vi "Validate Rate.vi"(8 "error IO":errorcluster, 9 "Ramping Mode":T1, 10 "rate":dbl[unit] caption="Rate", 11 "Power Supply in":refnum<class "Power Supply.lvclass">) -> (0 "error out":errorcluster, 1 "Max rate":dbl[unit], 2 "Coerced rate":dbl[unit], 3 "Power Supply out":refnum<class "Power Supply.lvclass">, 4 "Coerced?":bool, 6 "Field":dbl[unit])   [LabVIEW 2009, in "Power Supply.lvclass"]
doc: "Query the current field and verify that the given sweep rate is appropriate for this field."
uses:
  Power Supply.lvclass
  Ramping Mode.ctl
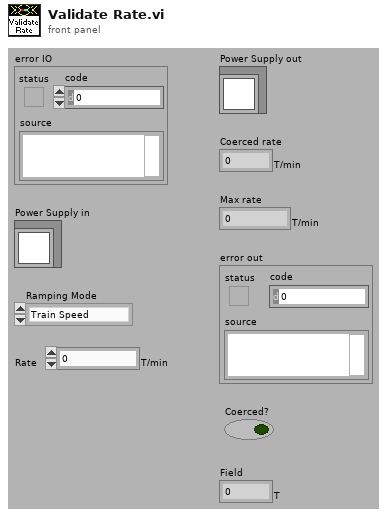
[diagram p1: front panel]
types:
  T1 = typedef "Power Supply.lvclass/Ramping Mode.ctl" = enum16{"Train Speed", "Maximum Speed", "Manual"}
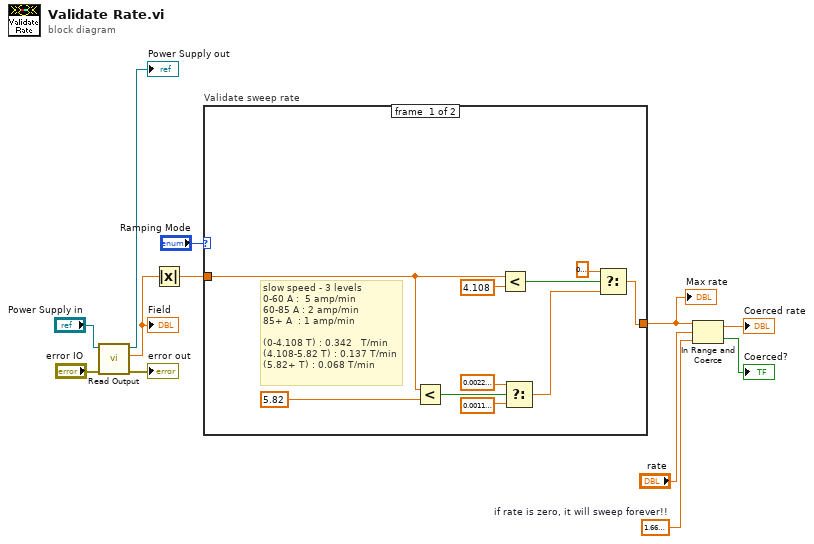
[diagram p0: block diagram]
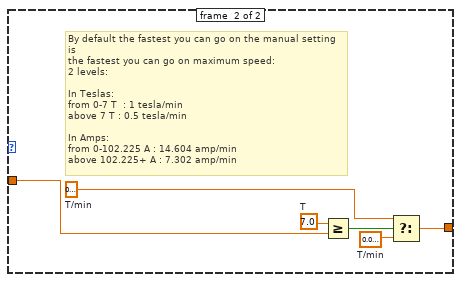
[diagram p2: hidden frame]
diagram:
  w6 = dbl[unit] 1.6666666666666667e-08  # if rate is zero, it will sweep forever!!
  n1 = call-dynamic "Read Output.vi"("error in (no error)"="error IO", "Power Supply in"="Power Supply in") -> ("error out"=→"error out":errorcluster, "Field"=w12:dbl[unit], "Power Supply out"=→"Power Supply out":refnum<class "Power Supply.lvclass">)  [unwired: 6 in, 1 out]
  "Field" <- w12
  n2 = Absolute Value(x=w12) -> (abs(x)=w2:dbl[unit])
  n3 = case "Validate sweep rate" shown="\"Train Speed\", Default" "Ramping Mode" {
    tunnel: w2 -> [w14 w23]
    tunnel: [w13 w24] -> w5
    frame #0 {
      # "slow speed - 3 levels\n0-60 A :  5 amp/min\n60-85 A : 2 amp/min\n85+ A  : 1 amp/min\n\n(0-4.108 T) : 0.342   T/min\n(4.108-5.82 T) : 0.137 T/min\n(5.82+ T) : 0.068 T/min"
      n4 = Less?(x=w14, y=dbl[unit] 5.82) -> (x < y?=w21:bool)
      n5 = Less?(x=w14, y=dbl[unit] 4.108) -> (x < y?=w15:bool)
      n6 = Select(t=dbl[unit] 0.0022833333333333334 ("y"), s=w21, f=dbl[unit] 0.0011333333333333334 ("y")) -> (s? t:f=w17:dbl[unit])
      n7 = Select(t=dbl[unit] 0.016666666666666666 ("y"), s=w15, f=w17) -> (s? t:f=w13:dbl[unit])
    }
    frame #1 {
      w26 = dbl[unit] 0.008333333333333333  # T/min
      w25 = dbl[unit] 0.016666666666666666  # T/min
      w27 = dbl[unit] 7.0  # T
      # "By default the fastest you can go on the manual setting is\nthe fastest you can go on maximum speed:\n2 levels:\n\nIn Teslas:\nfrom 0-7 T  : 1 tesla/min\nabove 7 T : 0.5 tesla/min\n\nIn Amps:\nfrom 0-102.225 A : 14.604 amp/min\nabove 102.225+ A : 7.302 amp/min"
      n8 = Greater Or Equal?(x=w27, y=w23) -> (x >= y?=w28:bool)
      n9 = Select(t=w25, s=w28, f=w26) -> (s? t:f=w24:dbl[unit])
    }
  }
  "Max rate" <- w5
  n10 = In Range and Coerce(upper limit=w5, x="rate", lower limit=w6) -> (coerced(x)=→"Coerced rate":dbl[unit], In Range?=→"Coerced?":bool)
